vi "Read Framework State Data.vi"(8 "error in (no error)":errorcluster, 11 "Framework Status in":refnum<class "Framework Status.lvclass">) -> (0 "error out":errorcluster, 2 "framework state data":T1 {"duration" format="%d us"}, 3 "Framework Status out":refnum<class "Framework Status.lvclass">)   [LabVIEW 2017, in "DSF Core.lvlib" / "Framework Status.lvclass"]
uses:
  Framework Status.lvclass
  Status/Status Data.ctl
  Framework Status.lvclass/Framework Status.ctl
  Status/Status Pointer.lvclass
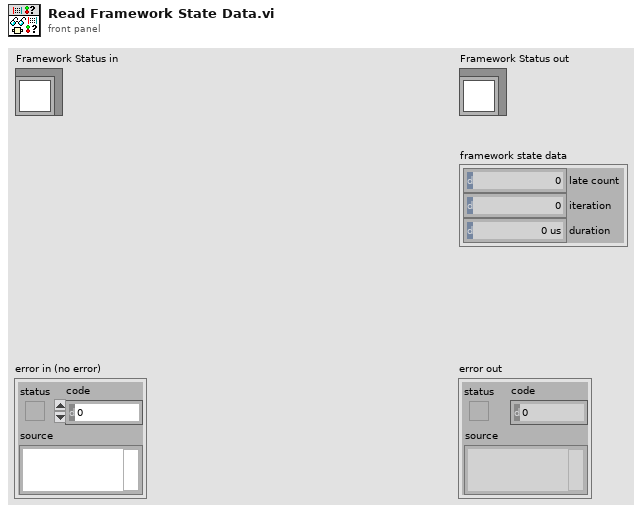
[diagram p1: front panel]
types:
  T1 = typedef "DSF Core.lvlib/Status Pointer.lvclass/Status Data.ctl" = cluster{"late count":u64, "iteration":u64, "duration":u32}
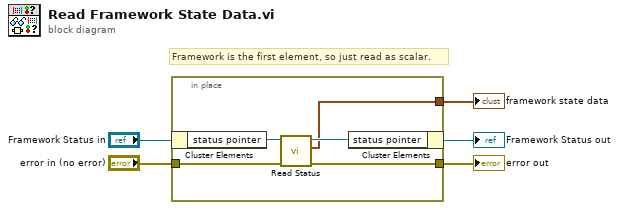
[diagram p0: block diagram]
diagram:
  # "Framework is the first element, so just read as scalar."
  n1 = in-place {
    in-place-border: "error in (no error)" -> [w8]
    in-place-border: [w7] -> w2
    in-place-border: [w6] -> w1
    n2 = in-place-cluster #1("Framework Status in") -> ("status pointer"=w10:refnum<class "Status Pointer.lvclass">)
    n3 = call "Read Status.vi"("error in (no error)"=w8, "status pointer in"=w10) -> ("error out"=w7:errorcluster, "status"=w6:T1, "status pointer out"=w9:refnum<class "Status Pointer.lvclass">)  [unwired: 7 in]
    n4 = in-place-cluster #1("status pointer"=w9) -> (→"Framework Status out":refnum<class "Framework Status.lvclass">)
  }
  "error out" <- w2
  "framework state data" <- w1
